vi "SignalGenerator.vi"(1 "Frequency":dbl, 2 "Amplitude":dbl) -> (8 "Waveform Graph":dynamicdata(graph))   [LabVIEW 2015]
doc: "SignalGenerator that generates a sine wave with given frequency and amplitude and outputs from AO 0."
panel:
  in  "Stop":bool
  out "Error Out":errorcluster
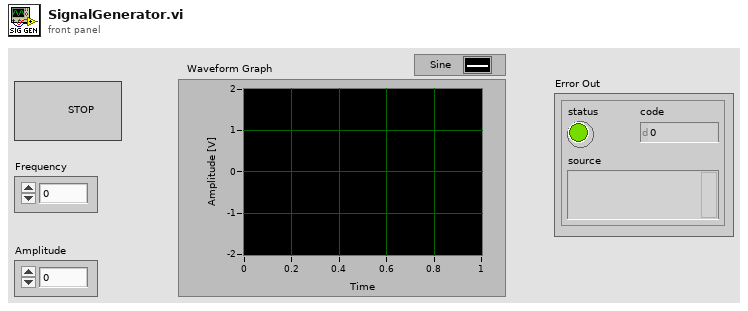
[diagram p1: front panel]
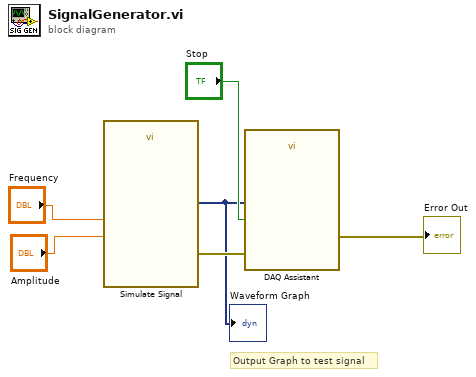
[diagram p0: block diagram]
diagram:
  # "Output Graph to test signal"
  n1 = call "Simulate Signal"("Frequency"="Frequency", "Amplitude"="Amplitude") -> ("Sine"=w3:dynamicdata, "error out"=w5:errorcluster)  [unwired: 12 in]
  "Waveform Graph" <- w3
  n2 = call "DAQ Assistant"("data"=w3, "error in"=w5, "stop (T)"="Stop") -> ("error out"=→"Error Out":errorcluster)  [unwired: 15 in, 1 out]
